vi "config_TRIG.vi"() -> ()   [LabVIEW 2011]
uses:
  global.vi
  <vilib>/Platform/browser.llb/Open URL in Default Browser (string).vi
panel:
  out "corrrected delay array":dbl[](array[numeric])=[0.0, 5.65e-06, 1.1e-06, 6.099999999999999e-06, 6.5999999999999995e-06, 4.66e-05, 6.399999999999999e-06, 1.1399999999999998e-05]
  out "Digital Waveform Graph":digitalwaveform(graph)={"t0"=timestamp(0 s since 1904-01-01), "dt"=1e-08, "Y"={"transitions"=[], "data"=array5126x5[25630 elements]}}
  in  "Burst":bool=TRUE
  in  "burst period":dbl=49.99999999999998 min=1e-07 format="%#_6f"
  in  "burst count":i32=3 min=2
  in  "duration":dbl[](array[numeric])=[5.65, 5.0, 40.0, 5.0] min=0.0 format="%.3f"
  in  "start time":dbl[](array[numeric])=[0.0, 1.1, 6.6000000000000005, 6.3999999999999995] format="%.3f"
  in  "time unit":enum16{"s", "ms", "us", "ns"}(ring)=enum."us"
  in  "Reset TRIG":bool
  in  "write config":bool
  in  "read delay data":bool
  in  "stop":bool
  in  "help":bool
  in  "AWG":bool=TRUE
  in  "SWITCH":bool
  in  "OSC":bool=TRUE
  in  "Power Amp":bool
  out "update front panel":bool
  # "Configure Delay Generator (TRIG)"
  # "power AMP"
  # "AWG"
  # "SWITCH"
  # "OSC"
  # "Polarity"
  # "NEGATIVE"
  # "POSITIVE"
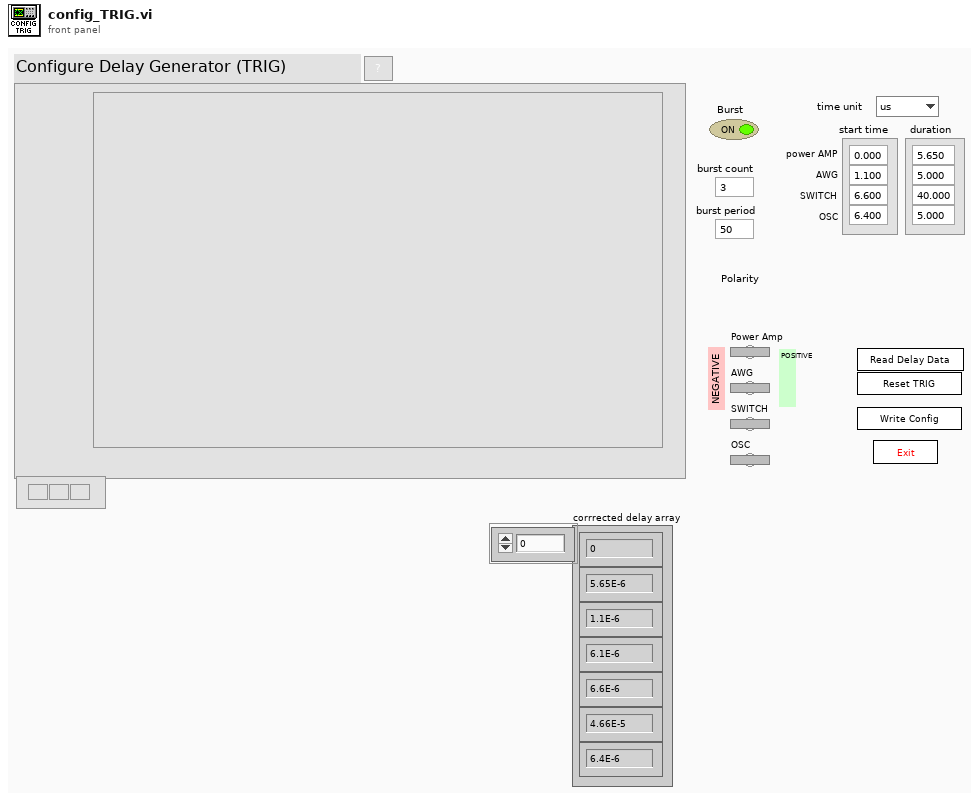
[diagram p1: front panel]
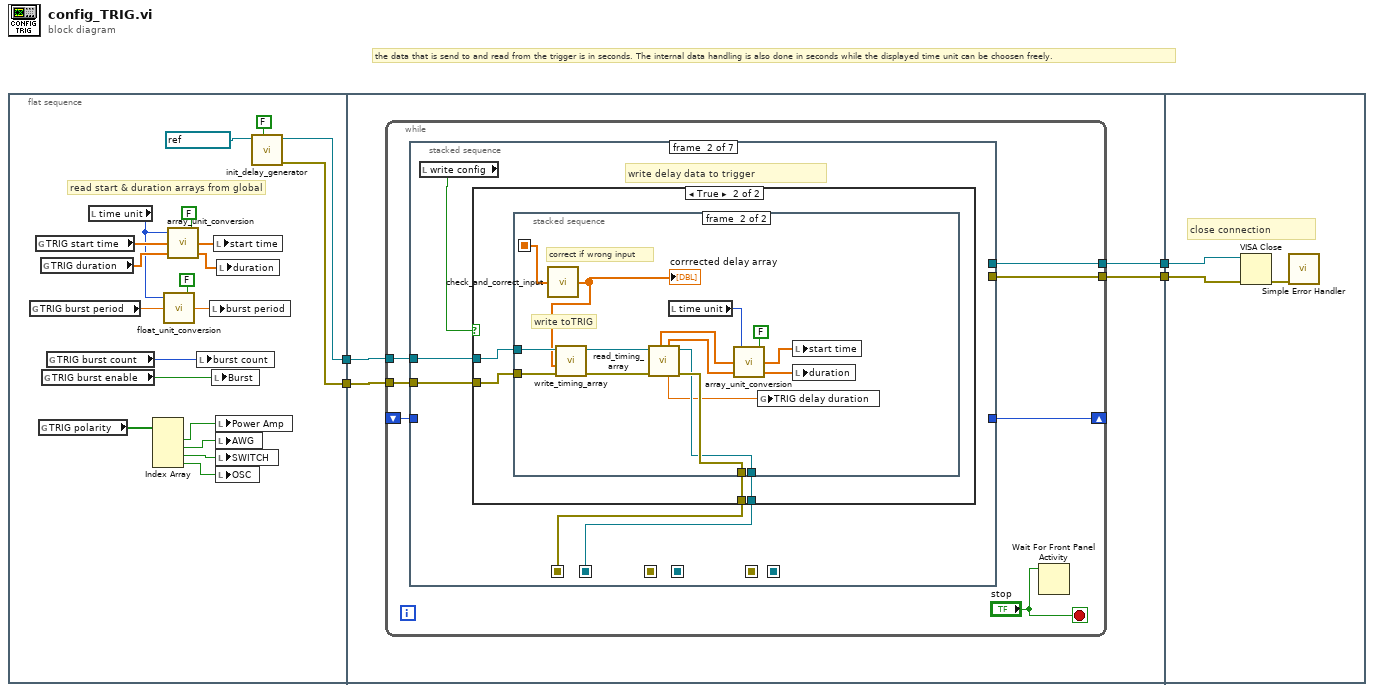
[diagram p0: block diagram]
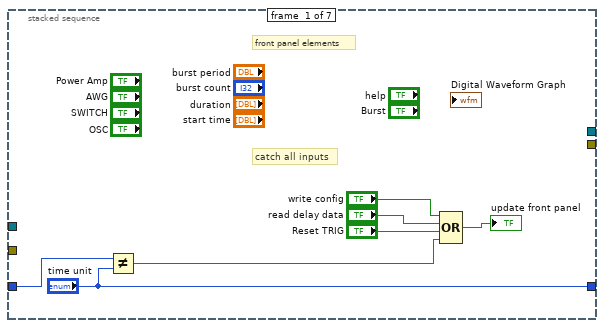
[diagram p2: hidden frame]
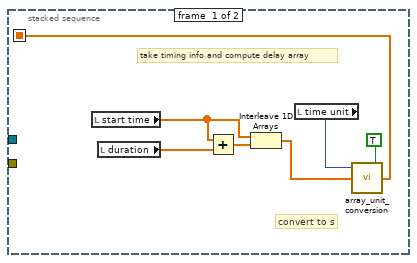
[diagram p4: hidden frame]
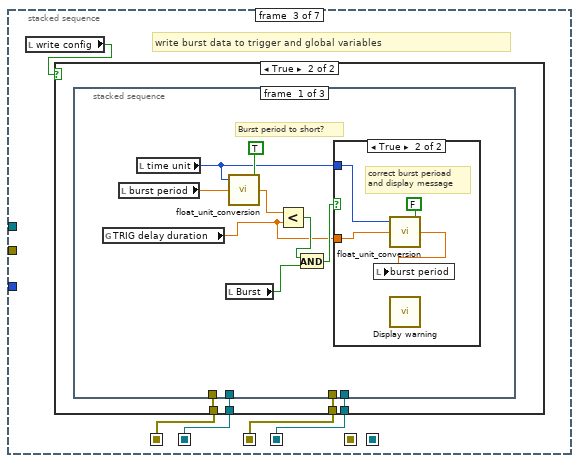
[diagram p5: hidden frame]
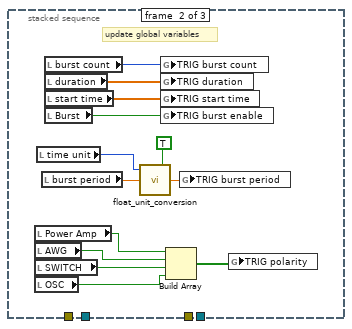
[diagram p8: hidden frame]
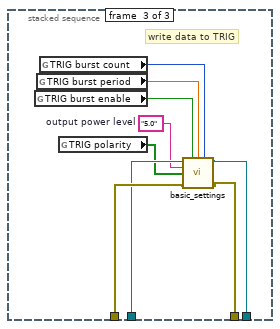
[diagram p9: hidden frame]
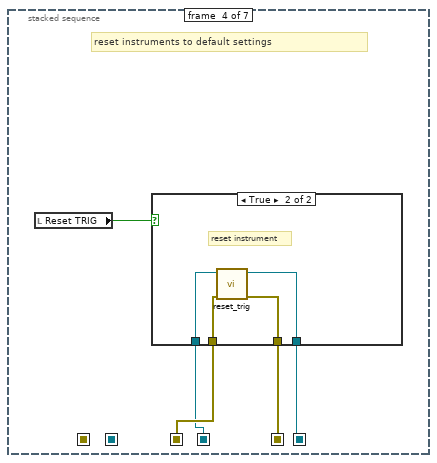
[diagram p10: hidden frame]
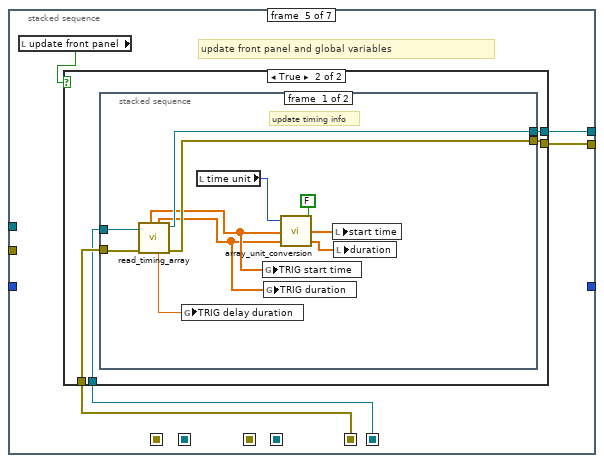
[diagram p12: hidden frame]
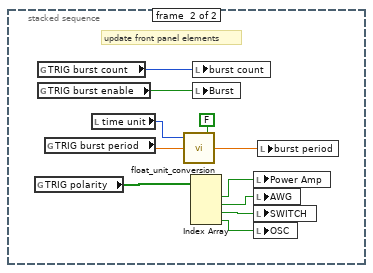
[diagram p14: hidden frame]
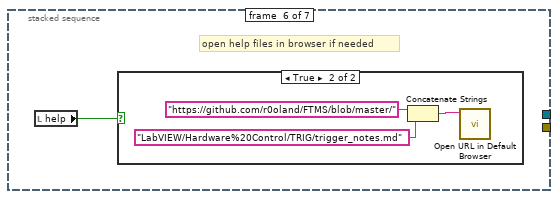
[diagram p15: hidden frame]
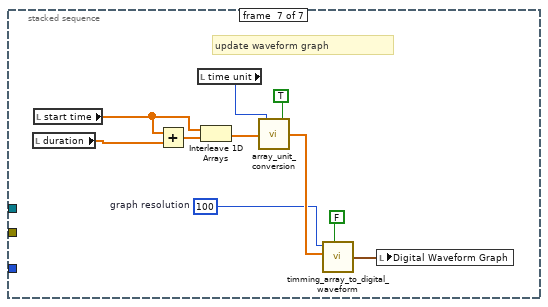
[diagram p17: hidden frame]
diagram:
  # "the data that is send to and read from the trigger is in seconds. The internal data handling is also done in seconds while the displayed time unit can be choosen freely."
  n1 = flat-sequence {
    tunnel: [w21] -> w2
    tunnel: [w20] -> w1
    tunnel: [w26] -> w4
    tunnel: [w25] -> w3
    tunnel: w2 -> [w28]
    tunnel: w1 -> [w27]
    tunnel: w4 -> [w181]
    tunnel: w3 -> [w180]
    frame #0 {
      # "read start & duration arrays from global"
      n2 = global read "global.vi" "TRIG burst period"() -> (w6:dbl)
      n3 = global read "global.vi" "TRIG start time"() -> (w19:dbl[])
      n4 = global read "global.vi" "TRIG polarity"() -> (w13:bool[])
      n5 = global read "global.vi" "TRIG duration"() -> (w17:dbl[])
      n6 = global read "global.vi" "TRIG burst enable"() -> (w14:bool)
      n7 = global read "global.vi" "TRIG burst count"() -> (w15:i32)
      n8 = local read "time unit"() -> (w5:enum16{"s", "ms", "us", "ns"})
      n9 = Index Array(array=w13) -> (element #1=w12:bool, element #2=w11:bool, element #3=w10:bool, element #4=w9:bool)  [unwired: 4 in]
      n10 = call "float_unit_conversion.vi"("inverse function (arb. unit to s)?"=FALSE, "time"=w6, "time unit"=w5) -> ("converted time"=w7:dbl)  [unwired: 2 in]
      n11 = call "array_unit_conversion.vi"("inverse function (arb. unit to s)?"=FALSE, "delay array 2"=w17, "delay array"=w19, "time unit"=w5) -> ("output 2"=w16:dbl[], "output"=w18:dbl[])
      n12 = local write "burst count"(w15) -> ()
      n13 = local write "burst period"(w7) -> ()
      n14 = local write "Burst"(w14) -> ()
      n15 = local write "start time"(w18) -> ()
      n16 = local write "Power Amp"(w12) -> ()
      n17 = local write "AWG"(w11) -> ()
      n18 = local write "SWITCH"(w10) -> ()
      n19 = local write "OSC"(w9) -> ()
      n20 = local write "duration"(w16) -> ()
      n21 = call "init_delay_generator.vi"("reset TRIG"=FALSE, "VISA resource name"=refnum<visa-resource-name> "TRIG2" ("TRIG2 resource name")) -> ("error out"=w20:errorcluster, "VISA resource name out"=w21:refnum<visa-resource-name>)  [unwired: 5 in]
    }
    frame #1 {
      n22 = while {
        tunnel: w27 -> [w33]
        tunnel: [w35] -> w26
        tunnel: [w34] -> w25
        tunnel: w28 -> [w31]
        shift-right: [w30] -> _
        shift-left: _ -> [w29]
        stop <- "stop" stop-if-true
        n23 = stacked-sequence {
          seq-local: [_ w43 _ _ _ _ _] -> [_ _ w79 _ _ _ _]
          seq-local: [_ w44 _ _ _ _ _] -> [_ _ w76 _ _ _ _]
          seq-local: [_ _ w77 _ _ _ _] -> [_ _ _ w125 _ _ _]
          seq-local: [_ _ w78 _ _ _ _] -> [_ _ _ w124 _ _ _]
          seq-local: [_ _ _ w121 _ _ _] -> [_ _ _ _ w135 _ _]
          seq-local: [_ _ _ w122 _ _ _] -> [_ _ _ _ w134 _ _]
          tunnel: w31 -> [_ w46 _ _ _ _ _]
          tunnel: w33 -> [_ w45 _ _ _ _ _]
          tunnel: [_ _ _ _ w133 _ _] -> w34
          tunnel: [_ _ _ _ w136 _ _] -> w35
          tunnel: ["time unit" _ _ _ _ _ _] -> w30
          tunnel: w29 -> [w37 _ _ _ _ _ _]
          frame #0 {
            # "front panel elements"
            # "catch all inputs"
            n24 = Not Equal?(x=w37, y="time unit") -> (x != y?=w38:bool)
            n25 = Compound Arithmetic op=OR("write config", "read delay data", "Reset TRIG", w38) -> (→"update front panel":bool)
          }
          frame #1 {
            # "write delay data to trigger"
            n26 = local read "write config"() -> (w47:bool)
            n27 = case shown="True" w47 {
              tunnel: w46 -> [w49 w53]
              tunnel: w45 -> [w48 w52]
              tunnel: [w49 w51] -> w44
              tunnel: [w48 w50] -> w43
              frame False {
              }
              frame True {
                n28 = stacked-sequence {
                  seq-local: [w56 _] -> [_ w71]
                  tunnel: w53 -> [_ w75]
                  tunnel: w52 -> [_ w74]
                  tunnel: [_ w68] -> w51
                  tunnel: [_ w69] -> w50
                  frame #0 {
                    # "convert to s"
                    # "take timing info and compute delay array"
                    n29 = local read "start time"() -> (w55:dbl[])
                    n30 = local read "duration"() -> (w54:dbl[])
                    n31 = Add(x=w55, y=w54) -> (x+y=w60:dbl[])
                    n32 = Interleave 1D Arrays(w55, w60) -> (w58:dbl[])
                    n33 = local read "time unit"() -> (w57:enum16{"s", "ms", "us", "ns"})
                    n34 = call "array_unit_conversion.vi"("inverse function (arb. unit to s)?"=TRUE, "delay array"=w58, "time unit"=w57) -> ("output"=w56:dbl[])  [unwired: 1 in, 1 out]
                  }
                  frame #1 {
                    # "write toTRIG"
                    # "correct if wrong input"
                    n35 = call "check_and_correct_input.vi"("delay array"=w71) -> ("corrrected delay array"=w70:dbl[])  [unwired: 4 in]
                    "corrrected delay array" <- w70
                    n36 = call "write_timing_array.vi"("error in"=w74, "delay array"=w70, "VISA resource in"=w75) -> ("error out 2"=w72:errorcluster, "VISA resource out"=w73:refnum<visa-resource-name>)  [unwired: 3 in]
                    n37 = call "read_timing_array.vi"("error in"=w72, "VISA resource in"=w73) -> ("error out 2"=w69:errorcluster, "VISA resource out"=w68:refnum<visa-resource-name>, "delay duration"=w61:dbl, "duration"=w65:dbl[], "start time"=w64:dbl[])  [unwired: 5 in]
                    n38 = local read "time unit"() -> (w66:enum16{"s", "ms", "us", "ns"})
                    n39 = call "array_unit_conversion.vi"("inverse function (arb. unit to s)?"=FALSE, "delay array 2"=w65, "delay array"=w64, "time unit"=w66) -> ("output 2"=w62:dbl[], "output"=w63:dbl[])
                    n40 = global write "global.vi" "TRIG delay duration"(w61) -> ()
                    n41 = local write "start time"(w63) -> ()
                    n42 = local write "duration"(w62) -> ()
                  }
                }
              }
            }
          }
          frame #2 {
            # "write burst data to trigger and global variables"
            n43 = local read "write config"() -> (w80:bool)
            n44 = case shown="True" w80 {
              tunnel: w79 -> [w81 w84]
              tunnel: w76 -> [w82 w83]
              tunnel: [w82 w86] -> w78
              tunnel: [w81 w85] -> w77
              frame False {
              }
              frame True {
                n45 = stacked-sequence {
                  tunnel: [_ _ w120] -> w86
                  tunnel: [_ _ w119] -> w85
                  tunnel: w84 -> [_ _ w118]
                  tunnel: w83 -> [_ _ w117]
                  frame #0 {
                    # "Burst period to short?"
                    n46 = global read "global.vi" "TRIG delay duration"() -> (w87:dbl)
                    n47 = local read "burst period"() -> (w93:dbl)
                    n48 = local read "time unit"() -> (w91:enum16{"s", "ms", "us", "ns"})
                    n49 = local read "Burst"() -> (w89:bool)
                    n50 = call "float_unit_conversion.vi"("inverse function (arb. unit to s)?"=TRUE, "time"=w93, "time unit"=w91) -> ("converted time"=w92:dbl)  [unwired: 2 in]
                    n51 = Less?(x=w92, y=w87) -> (x < y?=w90:bool)
                    n52 = And(x=w90, y=w89) -> (x .and. y?=w88:bool)
                    n53 = case shown="True" w88 {
                      tunnel: w91 -> [_ w97]
                      tunnel: w87 -> [_ w95]
                      frame False {
                      }
                      frame True {
                        # "correct burst perioad\nand display message"
                        n54 = call "float_unit_conversion.vi"("inverse function (arb. unit to s)?"=FALSE, "time"=w95, "time unit"=w97) -> ("converted time"=w96:dbl)  [unwired: 2 in]
                        n55 = local write "burst period"(w96) -> ()
                        n56 = call "Display warning"() -> ()  [unwired: 10 in, 2 out]
                      }
                    }
                  }
                  frame #1 {
                    # "update global variables"
                    n57 = local read "Power Amp"() -> (w100:bool)
                    n58 = local read "AWG"() -> (w101:bool)
                    n59 = local read "SWITCH"() -> (w102:bool)
                    n60 = local read "OSC"() -> (w103:bool)
                    n61 = local read "time unit"() -> (w99:enum16{"s", "ms", "us", "ns"})
                    n62 = local read "burst period"() -> (w111:dbl)
                    n63 = local read "burst count"() -> (w107:i32)
                    n64 = local read "duration"() -> (w108:dbl[])
                    n65 = local read "start time"() -> (w109:dbl[])
                    n66 = local read "Burst"() -> (w110:bool)
                    n67 = call "float_unit_conversion.vi"("inverse function (arb. unit to s)?"=TRUE, "time"=w111, "time unit"=w99) -> ("converted time"=w105:dbl)  [unwired: 2 in]
                    n68 = global write "global.vi" "TRIG burst count"(w107) -> ()
                    n69 = global write "global.vi" "TRIG duration"(w108) -> ()
                    n70 = global write "global.vi" "TRIG start time"(w109) -> ()
                    n71 = global write "global.vi" "TRIG burst enable"(w110) -> ()
                    n72 = Build Array(w100, w101, w102, w103) -> (w104:bool[])
                    n73 = global write "global.vi" "TRIG burst period"(w105) -> ()
                    n74 = global write "global.vi" "TRIG polarity"(w104) -> ()
                  }
                  frame #2 {
                    w113 = "5.0"  # output power level
                    # "write data to TRIG"
                    n75 = global read "global.vi" "TRIG burst enable"() -> (w114:bool)
                    n76 = global read "global.vi" "TRIG burst period"() -> (w115:dbl)
                    n77 = global read "global.vi" "TRIG burst count"() -> (w116:i32)
                    n78 = global read "global.vi" "TRIG polarity"() -> (w112:bool[])
                    n79 = call "basic_settings.vi"("VISA resource name"=w117, "Burst enable?"=w114, "burst period (s)"=w115, "burst count"=w116, "power level"=w113, "polarity"=w112, "error in (no error)"=w118) -> ("VISA resource name out"=w120:refnum<visa-resource-name>, "error out"=w119:errorcluster)  [unwired: 7 in]
                  }
                }
              }
            }
          }
          frame #3 {
            # "reset instruments to default settings"
            n80 = local read "Reset TRIG"() -> (w123:bool)
            n81 = case shown="True" w123 {
              tunnel: w125 -> [w126 w131]
              tunnel: w124 -> [w127 w130]
              tunnel: [w127 w128] -> w122
              tunnel: [w126 w129] -> w121
              frame False {
              }
              frame True {
                # "reset instrument"
                n82 = call "reset_trig.vi"("error in (no error)"=w131, "VISA resource name"=w130) -> ("error out"=w129:errorcluster, "VISA resource name out"=w128:refnum<visa-resource-name>)  [unwired: 8 in]
              }
            }
          }
          frame #4 {
            # "update front panel and global variables"
            n83 = local read "update front panel"() -> (w132:bool)
            n84 = case shown="True" w132 {
              tunnel: [w138 w142] -> w136
              tunnel: [w137 w141] -> w133
              tunnel: w135 -> [w137 w140]
              tunnel: w134 -> [w138 w139]
              frame False {
              }
              frame True {
                n85 = stacked-sequence {
                  tunnel: [w153 _] -> w142
                  tunnel: [w152 _] -> w141
                  tunnel: w140 -> [w151 _]
                  tunnel: w139 -> [w150 _]
                  frame #0 {
                    # "update timing info"
                    n86 = call "read_timing_array.vi"("error in"=w151, "VISA resource in"=w150) -> ("error out 2"=w152:errorcluster, "VISA resource out"=w153:refnum<visa-resource-name>, "delay duration"=w144:dbl, "duration"=w145:dbl[], "start time"=w146:dbl[])  [unwired: 5 in]
                    n87 = global write "global.vi" "TRIG delay duration"(w144) -> ()
                    n88 = local read "time unit"() -> (w143:enum16{"s", "ms", "us", "ns"})
                    n89 = global write "global.vi" "TRIG start time"(w146) -> ()
                    n90 = global write "global.vi" "TRIG duration"(w145) -> ()
                    n91 = call "array_unit_conversion.vi"("inverse function (arb. unit to s)?"=FALSE, "delay array 2"=w145, "delay array"=w146, "time unit"=w143) -> ("output 2"=w147:dbl[], "output"=w148:dbl[])
                    n92 = local write "start time"(w148) -> ()
                    n93 = local write "duration"(w147) -> ()
                  }
                  frame #1 {
                    # "update front panel elements"
                    n94 = global read "global.vi" "TRIG polarity"() -> (w163:bool[])
                    n95 = global read "global.vi" "TRIG burst count"() -> (w164:i32)
                    n96 = global read "global.vi" "TRIG burst enable"() -> (w162:bool)
                    n97 = global read "global.vi" "TRIG burst period"() -> (w160:dbl)
                    n98 = local read "time unit"() -> (w159:enum16{"s", "ms", "us", "ns"})
                    n99 = call "float_unit_conversion.vi"("inverse function (arb. unit to s)?"=FALSE, "time"=w160, "time unit"=w159) -> ("converted time"=w158:dbl)  [unwired: 2 in]
                    n100 = Index Array(array=w163) -> (element #1=w157:bool, element #2=w156:bool, element #3=w155:bool, element #4=w154:bool)  [unwired: 4 in]
                    n101 = local write "burst count"(w164) -> ()
                    n102 = local write "Burst"(w162) -> ()
                    n103 = local write "Power Amp"(w157) -> ()
                    n104 = local write "AWG"(w156) -> ()
                    n105 = local write "SWITCH"(w155) -> ()
                    n106 = local write "OSC"(w154) -> ()
                    n107 = local write "burst period"(w158) -> ()
                  }
                }
              }
            }
          }
          frame #5 {
            # "open help files in browser if needed"
            n108 = local read "help"() -> (w165:bool)
            n109 = case shown="True" w165 {
              frame False {
              }
              frame True {
                n110 = Concatenate Strings("https://github.com/r0oland/FTMS/blob/master/" ("string"), "LabVIEW/Hardware%20Control/TRIG/trigger_notes.md" ("string")) -> (w168:string)
                n111 = call-poly <vilib>:"Open URL in Default Browser.vi"("URL"=w168) -> ()  [unwired: 5 in, 2 out]
              }
            }
          }
          frame #6 {
            w174 = 100  # graph resolution
            # "update waveform graph"
            n112 = local read "duration"() -> (w171:dbl[])
            n113 = local read "start time"() -> (w172:dbl[])
            n114 = Add(x=w172, y=w171) -> (x+y=w178:dbl[])
            n115 = local read "time unit"() -> (w170:enum16{"s", "ms", "us", "ns"})
            n116 = Interleave 1D Arrays(w172, w178) -> (w176:dbl[])
            n117 = call "array_unit_conversion.vi"("inverse function (arb. unit to s)?"=TRUE, "delay array"=w176, "time unit"=w170) -> ("output"=w175:dbl[])  [unwired: 1 in, 1 out]
            n118 = call "timming_array_to_digital_waveform.vi"("resolution"=w174, "delay array"=w175, "Burst?"=FALSE) -> ("digital waveform"=w173:digitalwaveform)  [unwired: 3 in, 1 out]
            n119 = local write "Digital Waveform Graph"(w173) -> ()
          }
        }
        n120 = Wait For Front Panel Activity(3:"stop") -> ()  [unwired: 2 in, 1 out]
      }
    }
    frame #2 {
      # "close connection"
      n121 = VISA Close(VISA resource name=w181, error in (no error)=w180) -> (error out=w179:errorcluster)
      n122 = call <vilib>:"Simple Error Handler.vi"("error in (no error)"=w179) -> ()  [unwired: 4 in, 5 out]
    }
  }
